vi "S-BoxLookupArray.vi"(11 "In":u8[][](array[numeric])) -> (3 "Out":u8[][](array[numeric]))   [LabVIEW 2011, in "i3-external-encryption.lvlib"]
doc: "Perfoms the S-box lookup for a 2D-array.\n\n(c) Ton Plomp, 2011\nTHIS SOFTWARE IS PROVIDED AS IS, AND ANY WARRANTY IS REJECTED"
uses:
  i3-external-encryption.lvlib
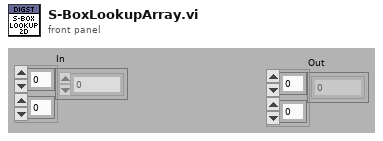
[diagram p1: front panel]
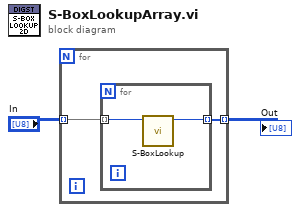
[diagram p0: block diagram]
diagram:
  n1 = for {
    tunnel: "In" -> [w4] mode=indexing
    tunnel: [w3] -> w1 mode=indexing
    n2 = for {
      tunnel: w4 -> [w6] mode=indexing
      tunnel: [w5] -> w3 mode=indexing
      n3 = call "S-BoxLookup.vi"("Value-In"=w6) -> ("LookUp-Out"=w5:u8)  [unwired: 10 in]
    }
  }
  "Out" <- w1
